vi "Send Auth Response.vi"(8 "error in (no error)":errorcluster, 10 "Response":T1, 11 "Connection in":refnum<class "Connection.lvclass">) -> (0 "error out":errorcluster, 1 "timeout":bool, 3 "Connection out":refnum<class "Connection.lvclass">)   [LabVIEW 2013, in "Connection_GOSPL.lvlib" / "Connection.lvclass"]
uses:
  Connection.lvclass
  auth response -- cluster.ctl
  Connection.lvclass/Connection.ctl
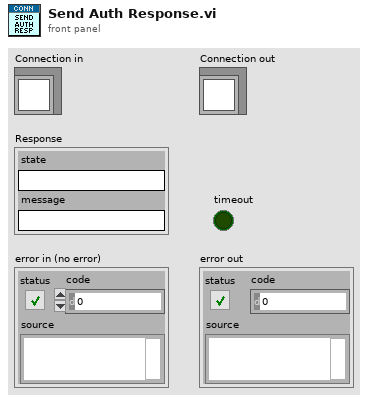
[diagram p1: front panel]
types:
  T1 = typedef "Connection_GOSPL.lvlib/Connection.lvclass/auth response -- cluster.ctl" = cluster{"state":string, "message":string}
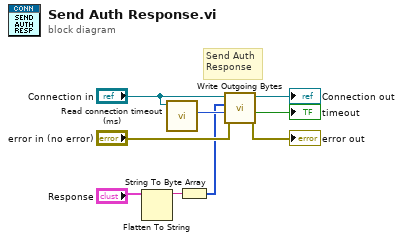
[diagram p0: block diagram]
diagram:
  # "Send Auth\nResponse"
  n1 = Flatten To String(anything="Response") -> (data string=w1:string)  [unwired: 3 in, 2 out]
  n2 = call "Read connection timeout (ms).vi"("Connection in"="Connection in") -> ("connection timeout (ms)"=w7:i32)  [unwired: 8 in, 2 out]
  n3 = String To Byte Array(string=w1) -> (unsigned byte array=w5:u8[])
  n4 = call-dynamic "Write Outgoing Bytes.vi"("error in (no error)"="error in (no error)", "timeout (2000 ms)"=w7, "Bytes"=w5, "Connection in"="Connection in") -> ("error out"=→"error out":errorcluster, "timeout"=→"timeout":bool, "Connection out"=→"Connection out":refnum<class "Connection.lvclass">)  [unwired: 5 in]
